vi "VISA Read TCP Hostname and Assert Valid.vi"(8 "error in":errorcluster, 10 "expected hostname":string, 11 "visa refnum in":refnum<visa-resource-name>) -> (0 "error out":errorcluster, 1 "result":string, 2 "pass?":bool, 3 "visa refnum out":refnum<visa-resource-name>)   [LabVIEW 2020, in "MeasurementServerTests.lvlib"]
uses:
  MeasurementServerTests.lvlib
  394c2a0e-59c1-4b09-b0dc-ca4f99f75ab1.vi
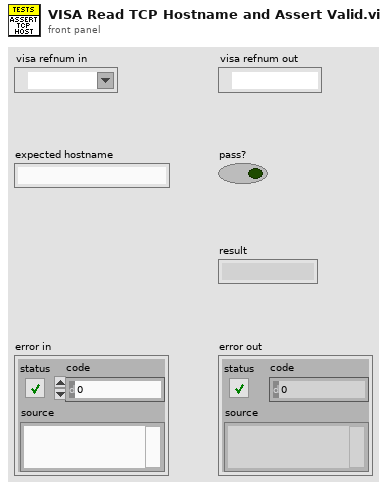
[diagram p1: front panel]
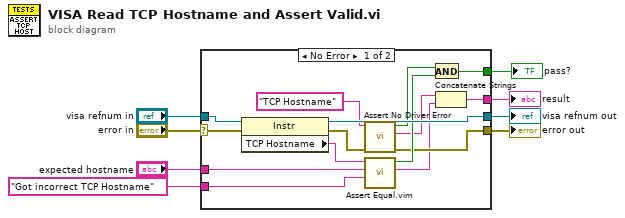
[diagram p0: block diagram]
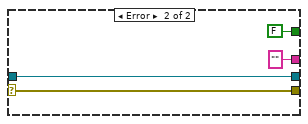
[diagram p2: hidden frame]
diagram:
  n1 = case shown="No Error" "error in" {
    selector: "error in" -> [w18 w26]
    tunnel: [w23 w27] -> w8
    tunnel: [w13 ""] -> w7
    tunnel: [w12 FALSE] -> w6
    tunnel: "Got incorrect TCP Hostname" ("failure message") -> [w21 _]
    tunnel: [w15 w26] -> w4
    tunnel: "visa refnum in" -> [w19 w27]
    tunnel: "expected hostname" -> [w17 _]
    frame No Error {
      n2 = property class="Instr"(reference=w19, error in=w18) -> (reference out=w23:refnum<visa-resource-name>, error out=w16:errorcluster, "TCP Hostname"=w20:string)
      n3 = call "Assert No Driver Error.vi"("error in"=w16, "driver vi name"="TCP Hostname") -> ("error out"=w15:errorcluster, "result"=w10:string, "pass?"=w11:bool)  [unwired: 7 in]
      n4 = call "Assert Equal.vim"("failure message"=w21, "actual value"=w17, "expected value"=w20) -> ("message"=w9:string, "equal?"=w22:bool)  [unwired: 7 in]
      n5 = And(x=w11, y=w22) -> (x .and. y?=w12:bool)
      n6 = Concatenate Strings(w10, w9) -> (w13:string)
    }
    frame Error {
    }
  }
  "visa refnum out" <- w8
  "result" <- w7
  "pass?" <- w6
  "error out" <- w4
